vi "INVALID SEQUENCE.vi"(0 "target_system":u8=6, 5 "target_component":u8=8) -> (4 "MAVLink Message":u8[](array[numeric]))   [LabVIEW 2014]
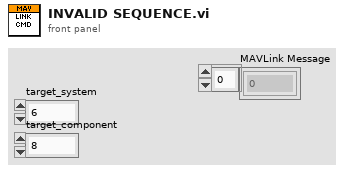
[diagram p1: front panel]
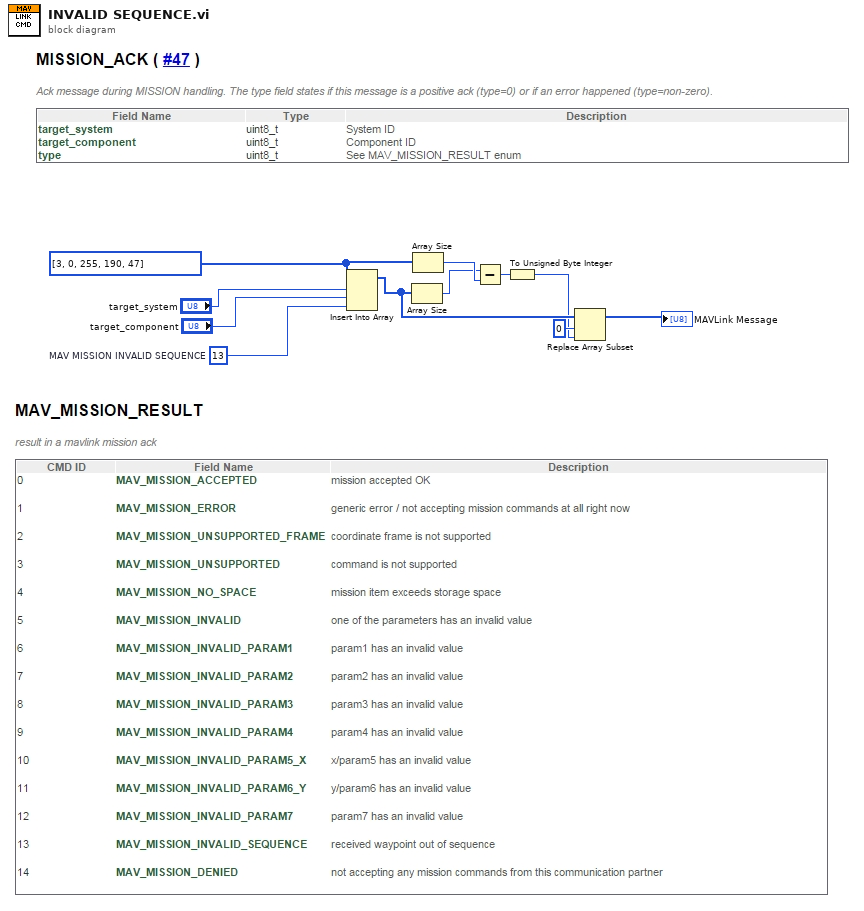
[diagram p0: block diagram]
diagram:
  w1 = u8 13  # MAV MISSION INVALID SEQUENCE
  w11 = u8[] [3, 0, 255, 190, 47]
  n1 = Insert Into Array(array=w11, index="target_system", new element #1="target_component", new element #2=w1) -> (w7:u8[])
  n2 = Array Size(array=w7) -> (size(s)=w9:i32)
  n3 = Array Size(array=w11) -> (size(s)=w10:i32)
  n4 = Subtract(x=w9, y=w10) -> (x-y=w8:i32)
  n5 = To Unsigned Byte Integer(number=w8) -> (unsigned 8bit integer=w5:u8)
  n6 = Replace Array Subset(array=w7, new element=w5, index=0) -> (→"MAVLink Message":u8[])
